vi "Pry.vi"(9 "force":dbl, 10 "Pryable in":refnum<class "Pryable.lvclass">, 11 "Lever in":refnum<class "Lever.lvclass">) -> (2 "Pryable out":refnum<class "Pryable.lvclass">)   [LabVIEW 2023, in "Lever.lvclass"]
uses:
  Lever.lvclass
  Pryable/Pryable.lvclass
panel:
  in  "force message":string="Force applied by %s:\n%f"
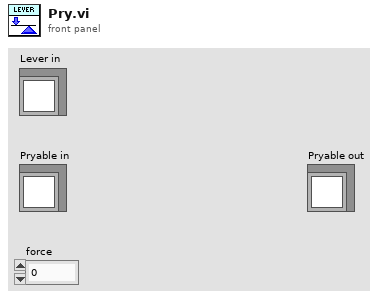
[diagram p1: front panel]
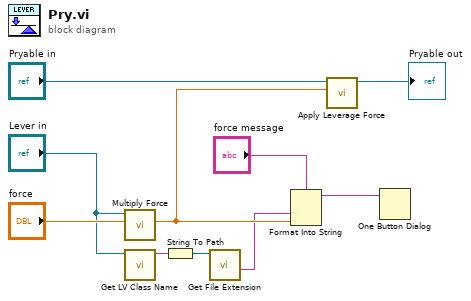
[diagram p0: block diagram]
diagram:
  n1 = call-dynamic "Multiply Force.vi"("force in"="force", "Lever in"="Lever in") -> ("force out"=w4:dbl)  [unwired: 9 in]
  n2 = call <vilib>:"Get LV Class Name.vi"("object"="Lever in") -> ("class name"=w3:string)  [unwired: 9 in, 1 out]
  n3 = String To Path(string=w3) -> (path=w2:path)
  n4 = call <vilib>:"Get File Extension.vi"("file"=w2) -> ("filename without extension"=w1:string)  [unwired: 6 in, 4 out]
  n5 = Format Into String(format string="force message", w1, w4) -> (resulting string=w7:string)  [unwired: 2 in, 1 out]
  n6 = call-dynamic "Apply Leverage Force.vi"("force"=w4, "Pryable in"="Pryable in") -> ("Pryable out"=→"Pryable out":refnum<class "Pryable.lvclass">)  [unwired: 9 in]
  n7 = One Button Dialog(message=w7) -> ()  [unwired: 1 in, 1 out]
